vi "DatastreamWrite.vi"(7 "Data":dbl[](array[numeric]), 8 "error in (no error)":errorcluster, 9 "port or service name":u16, 10 "address":u32, 11 "connection ID":refnum<k16>) -> (0 "error out":errorcluster, 3 "connection ID out":refnum<k16>)   [LabVIEW 2017]
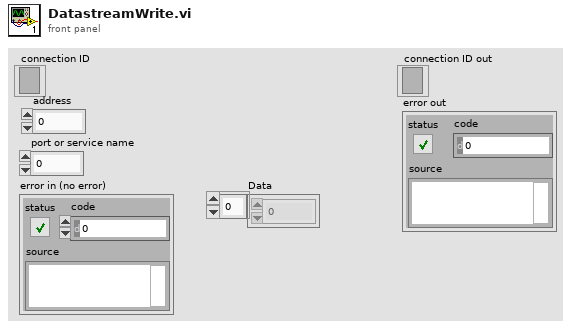
[diagram p1: front panel]
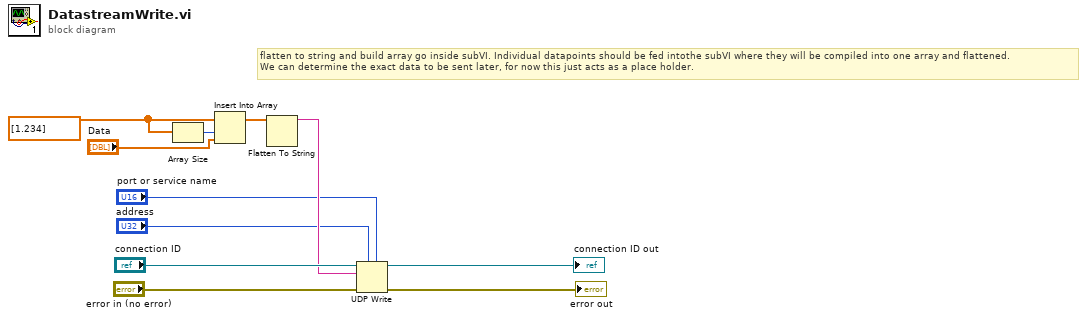
[diagram p0: block diagram]
diagram:
  w4 = dbl[] [1.234]
  # "flatten to string and build array go inside subVI. Individual datapoints should be fed intothe subVI where they will be compiled into one array and flattened. \nWe can determine the exact data to be sent later, for now this just acts as a place holder."
  n1 = Array Size(array=w4) -> (size(s)=w3:i32)
  n2 = Insert Into Array(array=w4, index=w3, new element="Data") -> (w1:dbl[])
  n3 = Flatten To String(anything=w1) -> (data string=w10:string)  [unwired: 3 in, 2 out]
  n4 = UDP Write(address="address", port or service name="port or service name", connection ID="connection ID", data in=w10, 8:"error in (no error)") -> (error out=→"error out":errorcluster, 3:→"connection ID out":refnum<k16>)  [unwired: 1 in]
